vi "Hardware Out - NI 9758-1 (PFI-LS).vi"(8 "RT Data in":T1={"Refs"={"FPGA 1"=refnum, "FPGA 2"=refnum}, "EPT"={"MaxCAD"=0.0, "EPT Sim Enabled"=FALSE, "EPTxData"={"Sync"=FALSE, "CurrentCAD"=0.0, "Speed [RPM]"=0.0, "Config"=FALSE, "Rcvg Primary"=FALSE, "Stall"=FALSE, "Overflow"=FALSE, "Ratio Error"=FALSE, "Pattern Error"=FALSE, "Aux Warning"=FALSE, "Watchdog Error"=FALSE}}, "Raw Inputs"={"NI9752s"=[], "NI9757s"=[], "NI9411s"=[], "NI9220s"=[], "VRHalls"=[]}, "Control Inputs"={"Engine Speed [RPM]"=0.0, "Engine Status"=enum."STALLED", "Load Control \nMode"=enum."High-Idle Governor", "dt(s)"=0.0, "Number of Cylinders"=0, "Engine Displacement [cc]"=0.0, "StoichAFR"=0.0, "Q.LHV Fuel [kJ/kg]"=0.0, "BattV PSU [V]"=0.0, "12V PSU [V]"=0.0, "5V PSU [V]"=0.0, "Pedal Position [%]"=0.0, "Oil Pressure [kPa]"=0.0, "Oil Temp [C]"=0.0, "Oil Level [%]"=0.0, "Engine Coolant Temp (ECT) [C]"=0.0, "Engine Coolant Pressure [kPa]"=0.0, "Rail Pressure [bar]"=0.0, "Fuel Pressure [kPa]"=0.0, "Fuel Temp [C]"=0.0, "Vacuum Pressure [kPa]"=0.0, "Throttle Position [%]"=0.0, "Cam1 Advance [CAD]"=0.0, "Cam2 Advance [CAD]"=0.0, "Cam3 Advance [CAD]"=0.0, "Cam4 Advance [CAD]"=0.0, "CA50 Control Output [CAD]"=[], "CA50 Control Output Valid"=[], "Intake Air Temp (IAT) [C]"=0.0, "Barometric Air Pressure [kPa]"=0.0, "Intake Air Rel. Humidity [%]"=0.0, "Mass Air Flow (MAF) [kg/hr]"=0.0, "Turbo Inlet Air Pressure [kPa]"=0.0, "Turbo Inlet Air Temp [C]"=0.0, "Turbo Outlet Air Pressure [kPa]"=0.0, "Turbo Outlet Air Temp [C]"=0.0, "CAC Outlet Pressure [kPa]"=0.0, "CAC Outlet Temp [C]"=0.0, "Intake Manifold Pressure (MAP) [kPa]"=0.0, "Intake Manifold Temp (MAT) [C]"=0.0, "Exhaust Manifold Pressure [kPa]"=0.0, "Exhaust Manifold Temp [C]"=0.0, "HighP EGR Cooler Outlet Pressure [kPa]"=0.0, "HighP EGR Cooler Outlet Temp [C]"=0.0, "HighP EGR Differential Pressure [kPa]"=0.0, "HighP EGR Valve Position [%]"=0.0, "Turbo Outlet Exhaust Pressure [kPa]"=0.0, "Turbo Outlet Exhaust Temp [C]"=0.0, "VGT Position 1 [%]"=0.0, "VGT Position 2 [%]"=0.0, "Turbo Speed 1 [RPM]"=0.0, "Turbo Speed 2 [RPM]"=0.0, "LowP EGR Differential Pressure [kPa]"=0.0, "LowP EGR Valve Position [%]"=0.0, "UEGO1Lambda"=0.0, "UEGO1_Hot"=FALSE, "UEGO2Lambda"=0.0, "UEGO2_Hot"=FALSE, "Knock Intensity"=[], "Knock"=[]}, "Control Outputs"={"Pedal Desired [%]"=0.0, "MEP Desired [bar]"=0.0, "Fuel Desired [mg/cyc]"=0.0, "Intake MAP Desired [kPa]"=0.0, "Cam1 Advance Setpoint [CAD]"=0.0, "Cam2 Advance Setpoint [CAD]"=0.0, "HighP EGR Position Setpoint [%Open]"=0.0, "LowP EGR Position Setpoint [%Open]"=0.0, "Rail Pressure Setpoint [bar]"=0.0, "Wastegate1 Position Setpoint [%Open]"=0.0, "Wastegate2 Position Setpoint [%Open]"=0.0, "VGT1 Position Setpoint [%Open]"=0.0, "VGT2 Position Setpoint [%Open]"=0.0, "Throttle1 Position Setpoint [%Open]"=0.0, "Throttle2 Position Setpoint [%Open]"=0.0, "TurboBPV Position Setpoint [%Open]"=0.0, "Spark Dwells [msec]"=[], "Spark Timings [DBTDC]"=[], "PFI Quantities [mg/inj]"=[], "PFI Timings [DBTDC]"=[], "DI Quantities [mg/inj]"=[], "DI Timings [DBTDC]"=[]}, "Raw Outputs"={"9751-1"={"DI1"={"Window_Start (DBTDC)"=0.0, "Window_End (DBTDC)"=0.0, "Enable_Inj1"=FALSE, "Duration_Inj1 (msec)"=0.0, "Timing_Inj1 (DBTDC)"=0.0, "Enable_Inj2"=FALSE, "Duration_Inj2 (msec)"=0.0, "Timing_Inj2 (DBTDC)"=0.0, "Enable_Inj3"=FALSE, "Duration_Inj3 (msec)"=0.0, "Timing_Inj3 (DBTDC)"=0.0, "Enable_Inj4"=FALSE, "Duration_Inj4 (msec)"=0.0, "Timing_Inj4 (DBTDC)"=0.0, "Enable_Inj5"=FALSE, "Duration_Inj5 (msec)"=0.0, "Timing_Inj5 (DBTDC)"=0.0}, "DI2"={"Window_Start (DBTDC)"=0.0, "Window_End (DBTDC)"=0.0, "Enable_Inj1"=FALSE, "Duration_Inj1 (msec)"=0.0, "Timing_Inj1 (DBTDC)"=0.0, "Enable_Inj2"=FALSE, "Duration_Inj2 (msec)"=0.0, "Timing_Inj2 (DBTDC)"=0.0, "Enable_Inj3"=FALSE, "Duration_Inj3 (msec)"=0.0, "Timing_Inj3 (DBTDC)"=0.0, "Enable_Inj4"=FALSE, "Duration_Inj4 (msec)"=0.0, "Timing_Inj4 (DBTDC)"=0.0, "Enable_Inj5"=FALSE, "Duration_Inj5 (msec)"=0.0, "Timing_Inj5 (DBTDC)"=0.0}, "DI3"={"Window_Start (DBTDC)"=0.0, "Window_End (DBTDC)"=0.0, "Enable_Inj1"=FALSE, "Duration_Inj1 (msec)"=0.0, "Timing_Inj1 (DBTDC)"=0.0, "Enable_Inj2"=FALSE, "Duration_Inj2 (msec)"=0.0, "Timing_Inj2 (DBTDC)"=0.0, "Enable_Inj3"=FALSE, "Duration_Inj3 (msec)"=0.0, "Timing_Inj3 (DBTDC)"=0.0, "Enable_Inj4"=FALSE, "Duration_Inj4 (msec)"=0.0, "Timing_Inj4 (DBTDC)"=0.0, "Enable_Inj5"=FALSE, "Duration_Inj5 (msec)"=0.0, "Timing_Inj5 (DBTDC)"=0.0}}, "9751-2"={"DI1"={"Window_Start (DBTDC)"=0.0, "Window_End (DBTDC)"=0.0, "Enable_Inj1"=FALSE, "Duration_Inj1 (msec)"=0.0, "Timing_Inj1 (DBTDC)"=0.0, "Enable_Inj2"=FALSE, "Duration_Inj2 (msec)"=0.0, "Timing_Inj2 (DBTDC)"=0.0, "Enable_Inj3"=FALSE, "Duration_Inj3 (msec)"=0.0, "Timing_Inj3 (DBTDC)"=0.0, "Enable_Inj4"=FALSE, "Duration_Inj4 (msec)"=0.0, "Timing_Inj4 (DBTDC)"=0.0, "Enable_Inj5"=FALSE, "Duration_Inj5 (msec)"=0.0, "Timing_Inj5 (DBTDC)"=0.0}, "DI2"={"Window_Start (DBTDC)"=0.0, "Window_End (DBTDC)"=0.0, "Enable_Inj1"=FALSE, "Duration_Inj1 (msec)"=0.0, "Timing_Inj1 (DBTDC)"=0.0, "Enable_Inj2"=FALSE, "Duration_Inj2 (msec)"=0.0, "Timing_Inj2 (DBTDC)"=0.0, "Enable_Inj3"=FALSE, "Duration_Inj3 (msec)"=0.0, "Timing_Inj3 (DBTDC)"=0.0, "Enable_Inj4"=FALSE, "Duration_Inj4 (msec)"=0.0, "Timing_Inj4 (DBTDC)"=0.0, "Enable_Inj5"=FALSE, "Duration_Inj5 (msec)"=0.0, "Timing_Inj5 (DBTDC)"=0.0}, "DI3"={"Window_Start (DBTDC)"=0.0, "Window_End (DBTDC)"=0.0, "Enable_Inj1"=FALSE, "Duration_Inj1 (msec)"=0.0, "Timing_Inj1 (DBTDC)"=0.0, "Enable_Inj2"=FALSE, "Duration_Inj2 (msec)"=0.0, "Timing_Inj2 (DBTDC)"=0.0, "Enable_Inj3"=FALSE, "Duration_Inj3 (msec)"=0.0, "Timing_Inj3 (DBTDC)"=0.0, "Enable_Inj4"=FALSE, "Duration_Inj4 (msec)"=0.0, "Timing_Inj4 (DBTDC)"=0.0, "Enable_Inj5"=FALSE, "Duration_Inj5 (msec)"=0.0, "Timing_Inj5 (DBTDC)"=0.0}}, "9751-3"={"DI1"={"Window_Start (DBTDC)"=0.0, "Window_End (DBTDC)"=0.0, "Enable_Inj1"=FALSE, "Duration_Inj1 (msec)"=0.0, "Timing_Inj1 (DBTDC)"=0.0, "Enable_Inj2"=FALSE, "Duration_Inj2 (msec)"=0.0, "Timing_Inj2 (DBTDC)"=0.0, "Enable_Inj3"=FALSE, "Duration_Inj3 (msec)"=0.0, "Timing_Inj3 (DBTDC)"=0.0, "Enable_Inj4"=FALSE, "Duration_Inj4 (msec)"=0.0, "Timing_Inj4 (DBTDC)"=0.0, "Enable_Inj5"=FALSE, "Duration_Inj5 (msec)"=0.0, "Timing_Inj5 (DBTDC)"=0.0}, "DI2"={"Window_Start (DBTDC)"=0.0, "Window_End (DBTDC)"=0.0, "Enable_Inj1"=FALSE, "Duration_Inj1 (msec)"=0.0, "Timing_Inj1 (DBTDC)"=0.0, "Enable_Inj2"=FALSE, "Duration_Inj2 (msec)"=0.0, "Timing_Inj2 (DBTDC)"=0.0, "Enable_Inj3"=FALSE, "Duration_Inj3 (msec)"=0.0, "Timing_Inj3 (DBTDC)"=0.0, "Enable_Inj4"=FALSE, "Duration_Inj4 (msec)"=0.0, "Timing_Inj4 (DBTDC)"=0.0, "Enable_Inj5"=FALSE, "Duration_Inj5 (msec)"=0.0, "Timing_Inj5 (DBTDC)"=0.0}, "DI3"={"Window_Start (DBTDC)"=0.0, "Window_End (DBTDC)"=0.0, "Enable_Inj1"=FALSE, "Duration_Inj1 (msec)"=0.0, "Timing_Inj1 (DBTDC)"=0.0, "Enable_Inj2"=FALSE, "Duration_Inj2 (msec)"=0.0, "Timing_Inj2 (DBTDC)"=0.0, "Enable_Inj3"=FALSE, "Duration_Inj3 (msec)"=0.0, "Timing_Inj3 (DBTDC)"=0.0, "Enable_Inj4"=FALSE, "Duration_Inj4 (msec)"=0.0, "Timing_Inj4 (DBTDC)"=0.0, "Enable_Inj5"=FALSE, "Duration_Inj5 (msec)"=0.0, "Timing_Inj5 (DBTDC)"=0.0}}, "9751-4"={"DI1"={"Window_Start (DBTDC)"=0.0, "Window_End (DBTDC)"=0.0, "Enable_Inj1"=FALSE, "Duration_Inj1 (msec)"=0.0, "Timing_Inj1 (DBTDC)"=0.0, "Enable_Inj2"=FALSE, "Duration_Inj2 (msec)"=0.0, "Timing_Inj2 (DBTDC)"=0.0, "Enable_Inj3"=FALSE, "Duration_Inj3 (msec)"=0.0, "Timing_Inj3 (DBTDC)"=0.0, "Enable_Inj4"=FALSE, "Duration_Inj4 (msec)"=0.0, "Timing_Inj4 (DBTDC)"=0.0, "Enable_Inj5"=FALSE, "Duration_Inj5 (msec)"=0.0, "Timing_Inj5 (DBTDC)"=0.0}, "DI2"={"Window_Start (DBTDC)"=0.0, "Window_End (DBTDC)"=0.0, "Enable_Inj1"=FALSE, "Duration_Inj1 (msec)"=0.0, "Timing_Inj1 (DBTDC)"=0.0, "Enable_Inj2"=FALSE, "Duration_Inj2 (msec)"=0.0, "Timing_Inj2 (DBTDC)"=0.0, "Enable_Inj3"=FALSE, "Duration_Inj3 (msec)"=0.0, "Timing_Inj3 (DBTDC)"=0.0, "Enable_Inj4"=FALSE, "Duration_Inj4 (msec)"=0.0, "Timing_Inj4 (DBTDC)"=0.0, "Enable_Inj5"=FALSE, "Duration_Inj5 (msec)"=0.0, "Timing_Inj5 (DBTDC)"=0.0}, "DI3"={"Window_Start (DBTDC)"=0.0, "Window_End (DBTDC)"=0.0, "Enable_Inj1"=FALSE, "Duration_Inj1 (msec)"=0.0, "Timing_Inj1 (DBTDC)"=0.0, "Enable_Inj2"=FALSE, "Duration_Inj2 (msec)"=0.0, "Timing_Inj2 (DBTDC)"=0.0, "Enable_Inj3"=FALSE, "Duration_Inj3 (msec)"=0.0, "Timing_Inj3 (DBTDC)"=0.0, "Enable_Inj4"=FALSE, "Duration_Inj4 (msec)"=0.0, "Timing_Inj4 (DBTDC)"=0.0, "Enable_Inj5"=FALSE, "Duration_Inj5 (msec)"=0.0, "Timing_Inj5 (DBTDC)"=0.0}}, "9754-1"={"ESTTL 1"={"Timing (DBTDC)"=0.0, "Dwell (ms)"=0.0}, "ESTTL 2"={"Timing (DBTDC)"=0.0, "Dwell (ms)"=0.0}, "ESTTL 3"={"Timing (DBTDC)"=0.0, "Dwell (ms)"=0.0}, "ESTTL 4"={"Timing (DBTDC)"=0.0, "Dwell (ms)"=0.0}, "ESTTL 5"={"Timing (DBTDC)"=0.0, "Dwell (ms)"=0.0}, "ESTTL 6"={"Timing (DBTDC)"=0.0, "Dwell (ms)"=0.0}, "ESTTL 7"={"Timing (DBTDC)"=0.0, "Dwell (ms)"=0.0}, "ESTTL 8"={"Timing (DBTDC)"=0.0, "Dwell (ms)"=0.0}}, "9754-2"={"ESTTL 1"={"Timing (DBTDC)"=0.0, "Dwell (ms)"=0.0}, "ESTTL 2"={"Timing (DBTDC)"=0.0, "Dwell (ms)"=0.0}, "ESTTL 3"={"Timing (DBTDC)"=0.0, "Dwell (ms)"=0.0}, "ESTTL 4"={"Timing (DBTDC)"=0.0, "Dwell (ms)"=0.0}, "ESTTL 5"={"Timing (DBTDC)"=0.0, "Dwell (ms)"=0.0}, "ESTTL 6"={"Timing (DBTDC)"=0.0, "Dwell (ms)"=0.0}, "ESTTL 7"={"Timing (DBTDC)"=0.0, "Dwell (ms)"=0.0}, "ESTTL 8"={"Timing (DBTDC)"=0.0, "Dwell (ms)"=0.0}}, "9758-1"={"LS 1"={"Enable"=FALSE, "Freq [Hz]"=0.0, "DutyCyc [%]"=0.0}, "LS 2"={"Enable"=FALSE, "Freq [Hz]"=0.0, "DutyCyc [%]"=0.0}, "LS 3"={"Enable"=FALSE, "Freq [Hz]"=0.0, "DutyCyc [%]"=0.0}, "LS 4"={"Enable"=FALSE, "Freq [Hz]"=0.0, "DutyCyc [%]"=0.0}, "PFI 1"={"Position Mode"=FALSE, "Timing (DBTDC)"=0.0, "Pulse Width (ms)"=0.0}, "PFI 2"={"Position Mode"=FALSE, "Timing (DBTDC)"=0.0, "Pulse Width (ms)"=0.0}, "PFI 3"={"Position Mode"=FALSE, "Timing (DBTDC)"=0.0, "Pulse Width (ms)"=0.0}, "PFI 4"={"Position Mode"=FALSE, "Timing (DBTDC)"=0.0, "Pulse Width (ms)"=0.0}}, "9758-2"={"LS 1"={"Enable"=FALSE, "Freq [Hz]"=0.0, "DutyCyc [%]"=0.0}, "LS 2"={"Enable"=FALSE, "Freq [Hz]"=0.0, "DutyCyc [%]"=0.0}, "LS 3"={"Enable"=FALSE, "Freq [Hz]"=0.0, "DutyCyc [%]"=0.0}, "LS 4"={"Enable"=FALSE, "Freq [Hz]"=0.0, "DutyCyc [%]"=0.0}, "PFI 1"={"Position Mode"=FALSE, "Timing (DBTDC)"=0.0, "Pulse Width (ms)"=0.0}, "PFI 2"={"Position Mode"=FALSE, "Timing (DBTDC)"=0.0, "Pulse Width (ms)"=0.0}, "PFI 3"={"Position Mode"=FALSE, "Timing (DBTDC)"=0.0, "Pulse Width (ms)"=0.0}, "PFI 4"={"Position Mode"=FALSE, "Timing (DBTDC)"=0.0, "Pulse Width (ms)"=0.0}}, "9759-1"={"THR1-1 DC [%]"=0.0, "THR1-1 Setpoint [% Open]"=0.0, "THR1-2 DC [%]"=0.0, "THR1-2 Setpoint [% Open]"=0.0}}} {"Control Inputs"."Knock Intensity" format="%.2f"; "Control Inputs"."CA50 Control Output [CAD]" format="%.2f"; "Control Inputs"."Exhaust Manifold Temp [C]" format="%#_6f"; "Control Inputs"."UEGO2Lambda" format="%.2f"; "Control Inputs"."Intake Manifold Temp (MAT) [C]" format="%#_6f"; "Control Inputs"."UEGO1Lambda" format="%.2f"}, 11 "FPGA Ref":T3) -> ()   [LabVIEW 2015, in "ECS-RT.lvlib"]
uses:
  ECS-RT.lvlib
  Typedefs/FPGA Refs/Generic FPGA Ref.ctl
  Typedefs/RT Data.ctl
  Typedefs/FPGA Refs/FPGA Refs.ctl
  Typedefs/EPT/EPT Cluster.ctl
  <vilib>/Powertrain Controls/Device Drivers/Engine Position Tracking/EPTx/RevA/RT/Controls/EPTxData.ctl
  Typedefs/Raw Inputs/Raw Inputs.ctl
  Typedefs/Raw Inputs/NI9752.ctl
  Typedefs/Raw Inputs/PPWData.ctl
  Typedefs/Raw Inputs/NI9757.ctl
  Typedefs/Raw Inputs/NI9411.ctl
  Typedefs/Raw Inputs/NI9220.ctl
  Typedefs/Raw Inputs/VRHall.ctl
  Typedefs/Control Inputs/Control Inputs.ctl
  Typedefs/EPT/Engine Status.ctl
  Typedefs/MISC/Load Control Mode.ctl
  Typedefs/Control Outputs/Control Outputs.ctl
  Typedefs/Control Outputs/Injection Quantity.ctl
  Typedefs/Control Outputs/Injection Timing.ctl
  Typedefs/Raw Outputs/Raw Outputs.ctl
  Typedefs/Raw Outputs/NI9751.ctl
  Typedefs/Raw Outputs/DI.ctl
  Typedefs/Raw Outputs/NI9754.ctl
  Typedefs/Raw Outputs/ESTTL.ctl
  Typedefs/Raw Outputs/NI9758.ctl
  Typedefs/Raw Outputs/LS.ctl
  Typedefs/Raw Outputs/PFI.ctl
  Typedefs/Raw Outputs/NI9759.ctl
  <vilib>/Powertrain Controls/Device Drivers/Engine Position Tracking/EPTx/RevA/RT/Controls/EPTxFuelSparkControl.ctl
  <vilib>/Utility/error.llb/Error Cluster From Error Code.vi
  <vilib>/rvi/errors/niLvFpgaAdjustHostInterfaceError.vi
  Globals/TDC Globals.vi
  <vilib>/rvi/interface/nirviReadWriteControl/nirviReadWriteControl.xnode
  <vilib>/rvi/interface/Simulation/niFpgaSimulationCallBeginRW.vi
  <vilib>/Powertrain Controls/Device Drivers/Engine Position Tracking/EPTx/RevA/RT/EPTx - RevA - RT.lvlib
  NiFpgaLv.dll
  ECS-Shared.lvlib
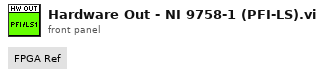
[diagram p1: front panel]
types:
  T1 = typedef "ECS-Shared.lvlib/RT Data.ctl" = cluster{"Refs":T2, "EPT":T4, "Raw Inputs":T6, "Control Inputs":T13, "Control Outputs":T16, "Raw Outputs":T19}
  T2 = typedef "ECS-Shared.lvlib/FPGA Refs.ctl" = cluster{"FPGA 1":T3, "FPGA 2":T3}
  T3 = typedef "ECS-Shared.lvlib/Generic FPGA Ref.ctl" = refnum<k20>
  T4 = typedef "ECS-Shared.lvlib/EPT Cluster.ctl" = cluster{"MaxCAD":sgl, "EPT Sim Enabled":bool, "EPTxData":T5}
  T5 = typedef "EPTx - RevA - RT.lvlib/EPTxData.ctl" = cluster{"Sync":bool, "CurrentCAD":sgl, "Speed [RPM]":sgl, "Config":bool, "Rcvg Primary":bool, "Stall":bool, "Overflow":bool, "Ratio Error":bool, "Pattern Error":bool, "Aux Warning":bool, "Watchdog Error":bool}
  T6 = typedef "ECS-Shared.lvlib/Raw Inputs.ctl" = cluster{"NI9752s":T7[], "NI9757s":T9[], "NI9411s":T10[], "NI9220s":T11[], "VRHalls":T12[]}
  T7 = typedef "ECS-Shared.lvlib/NI9752.ctl" = cluster{"Voltage [V]":sgl[], "Resistance [Ohm]":sgl[], "PPWData VR1":T8, "PPWData VR2":T8, "PPWData Hall1":T8, "PPWData Hall2":T8}
  T8 = typedef "ECS-Shared.lvlib/PPWData.ctl" = cluster{"Period":u32, "PulseWidth":u32, "Stopped":bool}
  T9 = typedef "ECS-Shared.lvlib/NI9757.ctl" = cluster{"UEGO1":cluster{"Lambda":sgl, "Phi":sgl, "AF_Ratio":sgl, "Ip":sgl, "Temp":sgl, "Hot":bool}, "UEGO2":cluster{"Lambda":sgl, "Phi":sgl, "AF_Ratio":sgl, "Ip":sgl, "Temp":sgl, "Hot":bool}, "EGO1":cluster{"Status":enum16{"COLD SENSOR", "FOULED SENSOR", "RICH", "LEAN"}, "SensorV":sgl}, "EGO2":cluster{"Status":enum16{"COLD SENSOR", "FOULED SENSOR", "RICH", "LEAN"}, "SensorV":sgl}, "EGO3":cluster{"Status":enum16{"COLD SENSOR", "FOULED SENSOR", "RICH", "LEAN"}, "SensorV":sgl}, "EGO4":cluster{"Status":enum16{"COLD SENSOR", "FOULED SENSOR", "RICH", "LEAN"}, "SensorV":sgl}}
  T10 = typedef "ECS-Shared.lvlib/NI9411.ctl" = cluster{"PPWData 0":T8, "PPWData 1":T8, "PPWData 2":T8, "PPWData 3":T8, "PPWData 4":T8, "PPWData 5":T8}
  T11 = typedef "ECS-Shared.lvlib/NI9220.ctl" = cluster{"AI 0":sgl, "AI 1":sgl, "AI 2":sgl, "AI 3":sgl, "AI 4":sgl, "AI 5":sgl, "AI 6":sgl, "AI 7":sgl, "AI 8":sgl, "AI 9":sgl, "AI 10":sgl, "AI 11":sgl, "AI 12":sgl, "AI 13":sgl, "AI 14":sgl, "AI 15":sgl}
  T12 = typedef "ECS-Shared.lvlib/VRHall.ctl" = cluster{"PPWData 0":T8, "PPWData 1":T8, "PPWData 2":T8, "PPWData 3":T8, "PPWData 4":T8, "PPWData 5":T8}
  T13 = typedef "ECS-Shared.lvlib/Control Inputs.ctl" = cluster{"Engine Speed [RPM]":sgl, "Engine Status":T14, "Load Control \nMode":T15, "dt(s)":sgl, "Number of Cylinders":u8, "Engine Displacement [cc]":sgl, "StoichAFR":sgl, "Q.LHV Fuel [kJ/kg]":sgl, "BattV PSU [V]":sgl, "12V PSU [V]":sgl, "5V PSU [V]":sgl, "Pedal Position [%]":sgl, "Oil Pressure [kPa]":sgl, "Oil Temp [C]":sgl, "Oil Level [%]":sgl, "Engine Coolant Temp (ECT) [C]":sgl, "Engine Coolant Pressure [kPa]":sgl, "Rail Pressure [bar]":sgl, "Fuel Pressure [kPa]":sgl, "Fuel Temp [C]":sgl, "Vacuum Pressure [kPa]":sgl, "Throttle Position [%]":sgl, "Cam1 Advance [CAD]":sgl, "Cam2 Advance [CAD]":sgl, "Cam3 Advance [CAD]":sgl, "Cam4 Advance [CAD]":sgl, "CA50 Control Output [CAD]":sgl[], "CA50 Control Output Valid":bool[], "Intake Air Temp (IAT) [C]":sgl, "Barometric Air Pressure [kPa]":sgl, "Intake Air Rel. Humidity [%]":sgl, "Mass Air Flow (MAF) [kg/hr]":sgl, "Turbo Inlet Air Pressure [kPa]":sgl, "Turbo Inlet Air Temp [C]":sgl, "Turbo Outlet Air Pressure [kPa]":sgl, "Turbo Outlet Air Temp [C]":sgl, "CAC Outlet Pressure [kPa]":sgl, "CAC Outlet Temp [C]":sgl, "Intake Manifold Pressure (MAP) [kPa]":sgl, "Intake Manifold Temp (MAT) [C]":sgl, "Exhaust Manifold Pressure [kPa]":sgl, "Exhaust Manifold Temp [C]":sgl, "HighP EGR Cooler Outlet Pressure [kPa]":sgl, "HighP EGR Cooler Outlet Temp [C]":sgl, "HighP EGR Differential Pressure [kPa]":sgl, "HighP EGR Valve Position [%]":sgl, "Turbo Outlet Exhaust Pressure [kPa]":sgl, "Turbo Outlet Exhaust Temp [C]":sgl, "VGT Position 1 [%]":sgl, "VGT Position 2 [%]":sgl, "Turbo Speed 1 [RPM]":sgl, "Turbo Speed 2 [RPM]":sgl, "LowP EGR Differential Pressure [kPa]":sgl, "LowP EGR Valve Position [%]":sgl, "UEGO1Lambda":sgl, "UEGO1_Hot":bool, "UEGO2Lambda":sgl, "UEGO2_Hot":bool, "Knock Intensity":sgl[], "Knock":bool[]}
  T14 = typedef "ECS-Shared.lvlib/Engine Status.ctl" = enum16{"OFF", "STALLED", "CRANKING", "RUNNING", "ACCEL", "DECEL", "SAFE"}
  T15 = typedef "ECS-Shared.lvlib/Load Control Mode.ctl" = enum16{"No Governor", "Low-Idle Governor", "High-Idle Governor"}
  T16 = typedef "ECS-Shared.lvlib/Control Outputs.ctl" = cluster{"Pedal Desired [%]":sgl, "MEP Desired [bar]":sgl, "Fuel Desired [mg/cyc]":sgl, "Intake MAP Desired [kPa]":sgl, "Cam1 Advance Setpoint [CAD]":sgl, "Cam2 Advance Setpoint [CAD]":sgl, "HighP EGR Position Setpoint [%Open]":sgl, "LowP EGR Position Setpoint [%Open]":sgl, "Rail Pressure Setpoint [bar]":sgl, "Wastegate1 Position Setpoint [%Open]":sgl, "Wastegate2 Position Setpoint [%Open]":sgl, "VGT1 Position Setpoint [%Open]":sgl, "VGT2 Position Setpoint [%Open]":sgl, "Throttle1 Position Setpoint [%Open]":sgl, "Throttle2 Position Setpoint [%Open]":sgl, "TurboBPV Position Setpoint [%Open]":sgl, "Spark Dwells [msec]":sgl[], "Spark Timings [DBTDC]":sgl[], "PFI Quantities [mg/inj]":sgl[], "PFI Timings [DBTDC]":sgl[], "DI Quantities [mg/inj]":T17[], "DI Timings [DBTDC]":T18[]}
  T17 = typedef "ECS-Shared.lvlib/Injection Quantity.ctl" = cluster{"Pilot1Quantity [mg/inj]":sgl, "Pilot2Quantity [mg/inj]":sgl, "MainQuantity [mg/inj]":sgl, "Post1Quantity [mg/inj]":sgl, "Post2Quantity [mg/inj]":sgl}
  T18 = typedef "ECS-Shared.lvlib/Injection Timing.ctl" = cluster{"Pilot1SOI [DBTDC]":sgl, "Pilot2SOI [DBTDC]":sgl, "MainSOI [DBTDC]":sgl, "Post1SOI [DBTDC]":sgl, "Post2SOI [DBTDC]":sgl}
  T19 = typedef "ECS-Shared.lvlib/Raw Outputs.ctl" = cluster{"9751-1":T20, "9751-2":T20, "9751-3":T20, "9751-4":T20, "9754-1":T22, "9754-2":T22, "9758-1":T24, "9758-2":T24, "9759-1":T27}
  T20 = typedef "ECS-Shared.lvlib/NI9751.ctl" = cluster{"DI1":T21, "DI2":T21, "DI3":T21}
  T21 = typedef "ECS-Shared.lvlib/DI.ctl" = cluster{"Window_Start (DBTDC)":sgl, "Window_End (DBTDC)":sgl, "Enable_Inj1":bool, "Duration_Inj1 (msec)":sgl, "Timing_Inj1 (DBTDC)":sgl, "Enable_Inj2":bool, "Duration_Inj2 (msec)":sgl, "Timing_Inj2 (DBTDC)":sgl, "Enable_Inj3":bool, "Duration_Inj3 (msec)":sgl, "Timing_Inj3 (DBTDC)":sgl, "Enable_Inj4":bool, "Duration_Inj4 (msec)":sgl, "Timing_Inj4 (DBTDC)":sgl, "Enable_Inj5":bool, "Duration_Inj5 (msec)":sgl, "Timing_Inj5 (DBTDC)":sgl}
  T22 = typedef "ECS-Shared.lvlib/NI9754.ctl" = cluster{"ESTTL 1":T23, "ESTTL 2":T23, "ESTTL 3":T23, "ESTTL 4":T23, "ESTTL 5":T23, "ESTTL 6":T23, "ESTTL 7":T23, "ESTTL 8":T23}
  T23 = typedef "ECS-Shared.lvlib/ESTTL.ctl" = cluster{"Timing (DBTDC)":sgl, "Dwell (ms)":sgl}
  T24 = typedef "ECS-Shared.lvlib/NI9758.ctl" = cluster{"LS 1":T25, "LS 2":T25, "LS 3":T25, "LS 4":T25, "PFI 1":T26, "PFI 2":T26, "PFI 3":T26, "PFI 4":T26}
  T25 = typedef "ECS-Shared.lvlib/LS.ctl" = cluster{"Enable":bool, "Freq [Hz]":sgl, "DutyCyc [%]":sgl}
  T26 = typedef "ECS-Shared.lvlib/PFI.ctl" = cluster{"Position Mode":bool, "Timing (DBTDC)":sgl, "Pulse Width (ms)":sgl}
  T27 = typedef "ECS-Shared.lvlib/NI9759.ctl" = cluster{"THR1-1 DC [%]":sgl, "THR1-1 Setpoint [% Open]":sgl, "THR1-2 DC [%]":sgl, "THR1-2 Setpoint [% Open]":sgl}
  T28 = typedef "EPTx - RevA - RT.lvlib/EPTxFuelSparkControl.ctl" = cluster{"Enable":bool, "Window Start [DBTDC]":sgl, "Window End [DBTDC]":sgl, "Timing [DBTDC]":sgl, "Duration [ms]":sgl, "Timing Mode (SA=F, EA=T)":bool, "Min Duration [ms]":sgl, "Max Duration [ms]":sgl}
  T29 = cluster{"LS1Period":u32, "LS1PulseWidth":u32, "LS2Period":u32, "LS2PulseWidth":u32, "LS3Period":u32, "LS3PulseWidth":u32, "LS4Period":u32, "LS4PulseWidth":u32}
  T30 = cluster{"ModuleEnable":bool, "LS1Enable":bool, "LS2Enable":bool, "LS3Enable":bool, "LS4Enable":bool, "PFI1Enable":bool, "PFI2Enable":bool, "PFI3Enable":bool, "PFI4Enable":bool, "RecircAlways1":bool, "RecircAlways2":bool, "RecircAlways3":bool, "RecircAlways4":bool, "Phase1FirstPeak1":bool, "Phase1FirstPeak2":bool, "Phase1FirstPeak3":bool, "Phase1FirstPeak4":bool, "OneShotSelect":enum8{"DISABLED", "PFI 1", "PFI 2", "PFI 3", "PFI 4"}, "One Shot Time (msec)":sgl, "OneShot":bool, "Fault_ClrSig":bool}
  T31 = cluster{"IPhaseCurrent":u16, "IPhaseDuration":u16}[]
  T32 = typedef "EPTx - RevA - FPGA.lvlib/EPTxFuelSparkControl.ctl" = cluster{"Enable":bool, "Window Start [CAD]":fxp<+,18,11>, "Window End [CAD]":fxp<+,18,11>, "Timing [CAD]":fxp<+,18,11>, "Duration [ms]":fxp<+/-,22,9>}
  T33 = cluster{"ModuleEnable":bool, "WatchdogIn":bool, "OneShotSelect":enum8{"DISABLED", "PFI 1", "PFI 2", "PFI 3", "PFI 4"}, "OneShotTime":u32, "OneShot":bool, "Control":u16, "HostMode":u8, "HostCommand":u32, "Fault_ClrSig":bool}
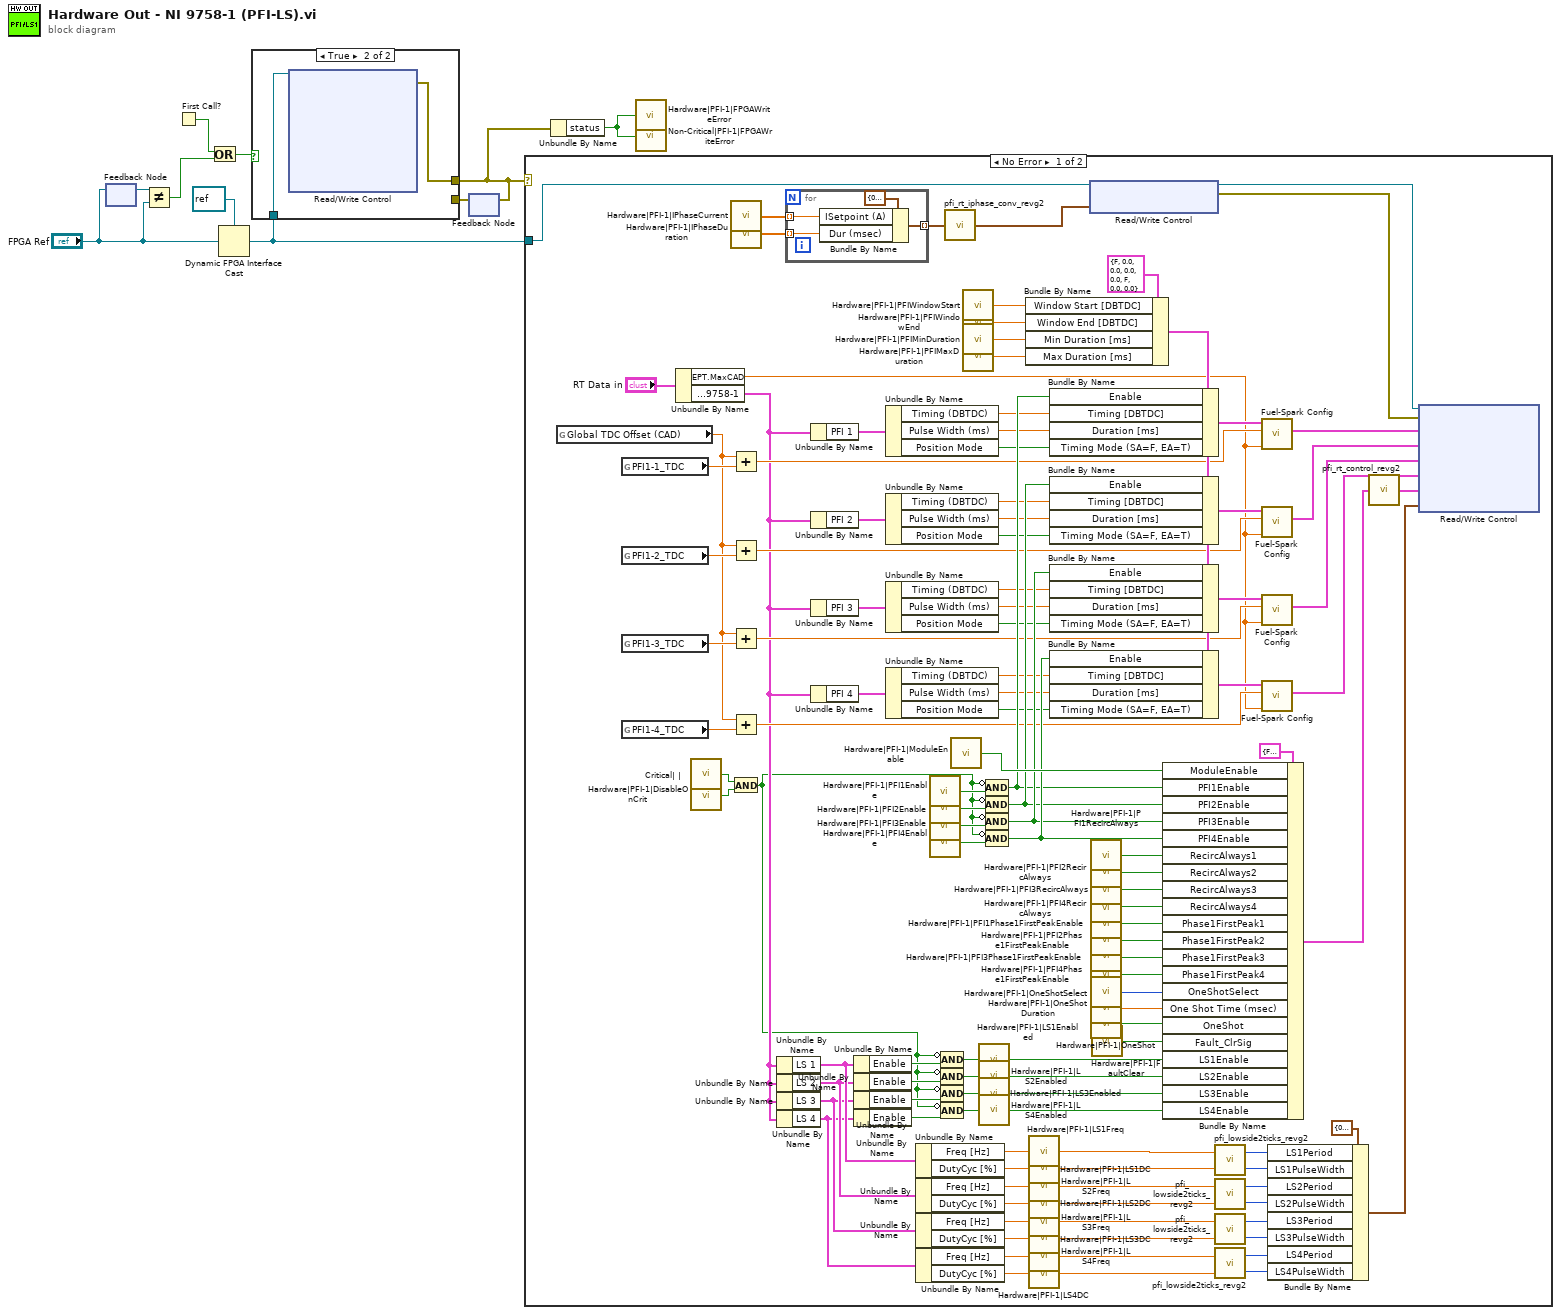
[diagram p0: block diagram]
diagram:
  n1 = feedback #1() -> (w7:T3)  [unwired: 1 in]
  n2 = feedback-in #1("FPGA Ref") -> ()
  n3 = Not Equal?(x=w7, y="FPGA Ref") -> (x != y?=w6:bool)
  n4 = First Call?() -> (First Call?: T/F=w8:bool)
  n5 = Or(x=w8, y=w6) -> (x .or. y?=w9:bool)
  n6 = Dynamic FPGA Interface Cast(Session In=refnum<k20> refnum ("NI 9758-1 (PFI-LS)"), Type="FPGA Ref") -> (Session Out=w3:refnum<k20>)
  n7 = feedback #2() -> (w10:errorcluster)  [unwired: 1 in]
  n8 = case shown="True" w9 {
    tunnel: [w11 w13] -> w2
    tunnel: w10 -> [w11 _]
    tunnel: w3 -> [_ w12]
    frame False {
    }
    frame True {
      n9 = xnode "Read/Write Control"("FPGA VI Reference In"=w12) -> ("error out"=w13:errorcluster)  [unwired: 8 in, 1 out]
    }
  }
  n10 = feedback-in #2(w2) -> ()
  n11 = case shown="No Error" w2 {
    tunnel: w3 -> [w63 _]
    frame No Error {
      n12 = global read "TDC Globals.vi" "Global TDC Offset (CAD)"() -> (w62:sgl)
      n13 = global read "TDC Globals.vi" "PFI1-1_TDC"() -> (w66:sgl)
      n14 = global read "TDC Globals.vi" "PFI1-2_TDC"() -> (w67:sgl)
      n15 = global read "TDC Globals.vi" "PFI1-3_TDC"() -> (w68:sgl)
      n16 = global read "TDC Globals.vi" "PFI1-4_TDC"() -> (w69:sgl)
      n17 = Unbundle By Name("RT Data in") -> ("EPT.MaxCAD"=w22:sgl, "Raw Outputs.9758-1"=w21:T24)
      n18 = call "Critical| |"() -> ("Fault"=w16:bool)  [unwired: 2 in]
      n19 = call "Hardware|PFI-1|DisableOnCrit"() -> ("Value"=w15:bool)
      n20 = call "Hardware|PFI-1|IPhaseCurrent"() -> ("Value"=w77:sgl[])
      n21 = call "Hardware|PFI-1|IPhaseDuration"() -> ("Value"=w78:sgl[])
      n22 = Add(x=w62, y=w66) -> (x+y=w31:sgl)
      n23 = Add(x=w62, y=w67) -> (x+y=w30:sgl)
      n24 = Add(x=w62, y=w68) -> (x+y=w29:sgl)
      n25 = Add(x=w62, y=w69) -> (x+y=w28:sgl)
      n26 = And(x=w16, y=w15) -> (x .and. y?=w14:bool)
      n27 = Unbundle By Name(w21) -> ("LS 1"=w20:T25)
      n28 = Unbundle By Name(w21) -> ("LS 2"=w19:T25)
      n29 = Unbundle By Name(w21) -> ("LS 3"=w18:T25)
      n30 = Unbundle By Name(w21) -> ("LS 4"=w17:T25)
      n31 = for {
        tunnel: w77 -> [w123] mode=indexing
        tunnel: w78 -> [w122] mode=indexing
        tunnel: [w121] -> w79 mode=indexing
        n32 = Bundle By Name(cluster=cluster{"ISetpoint (A)":sgl, "Dur (msec)":sgl} {"ISetpoint (A)"=0.0, "Dur (msec)"=0.0} ("IPhaseInterface"), "ISetpoint (A)"=w123, "Dur (msec)"=w122) -> (w121:cluster{"ISetpoint (A)":sgl, "Dur (msec)":sgl})
      }
      n33 = Unbundle By Name(w21) -> ("PFI 1"=w27:T26)
      n34 = Unbundle By Name(w21) -> ("PFI 2"=w25:T26)
      n35 = Unbundle By Name(w21) -> ("PFI 3"=w24:T26)
      n36 = Unbundle By Name(w21) -> ("PFI 4"=w23:T26)
      n37 = Unbundle By Name(w20) -> ("Enable"=w118:bool)
      n38 = Unbundle By Name(w19) -> ("Enable"=w119:bool)
      n39 = Unbundle By Name(w18) -> ("Enable"=w95:bool)
      n40 = Unbundle By Name(w17) -> ("Enable"=w94:bool)
      n41 = Unbundle By Name(w27) -> ("Timing (DBTDC)"=w43:sgl, "Pulse Width (ms)"=w42:sgl, "Position Mode"=w41:bool)
      n42 = Unbundle By Name(w25) -> ("Timing (DBTDC)"=w40:sgl, "Pulse Width (ms)"=w39:sgl, "Position Mode"=w38:bool)
      n43 = Unbundle By Name(w24) -> ("Timing (DBTDC)"=w37:sgl, "Pulse Width (ms)"=w36:sgl, "Position Mode"=w35:bool)
      n44 = Unbundle By Name(w23) -> ("Timing (DBTDC)"=w34:sgl, "Pulse Width (ms)"=w33:sgl, "Position Mode"=w32:bool)
      n45 = Unbundle By Name(w20) -> ("Freq [Hz]"=w87:sgl, "DutyCyc [%]"=w86:sgl)
      n46 = Unbundle By Name(w19) -> ("Freq [Hz]"=w85:sgl, "DutyCyc [%]"=w84:sgl)
      n47 = Unbundle By Name(w18) -> ("Freq [Hz]"=w83:sgl, "DutyCyc [%]"=w82:sgl)
      n48 = Unbundle By Name(w17) -> ("Freq [Hz]"=w81:sgl, "DutyCyc [%]"=w80:sgl)
      n49 = call "Hardware|PFI-1|PFI1Enable"() -> ("Value"=w113:bool)
      n50 = call "Hardware|PFI-1|PFI2Enable"() -> ("Value"=w114:bool)
      n51 = call "Hardware|PFI-1|PFI3Enable"() -> ("Value"=w115:bool)
      n52 = call "Hardware|PFI-1|PFI4Enable"() -> ("Value"=w116:bool)
      n53 = Compound Arithmetic op=AND(invert w14, w118) -> (w75:bool)
      n54 = Compound Arithmetic op=AND(invert w14, w119) -> (w74:bool)
      n55 = Compound Arithmetic op=AND(invert w14, w95) -> (w73:bool)
      n56 = Compound Arithmetic op=AND(invert w14, w94) -> (w72:bool)
      n57 = call <vilib>:"pfi_rt_iphase_conv_revg2.vi"("IPhaseArrayIn"=w79) -> ("IPhaseArrayOut"=w76:T31)
      n58 = call "Hardware|PFI-1|ModuleEnable"() -> ("Value"=w117:bool)
      n59 = call "Hardware|PFI-1|PFIWindowStart"() -> ("Value"=w48:sgl)
      n60 = call "Hardware|PFI-1|PFIWindowEnd"() -> ("Value"=w47:sgl)
      n61 = call "Hardware|PFI-1|PFIMinDuration"() -> ("Value"=w45:sgl)
      n62 = call "Hardware|PFI-1|PFIMaxDuration"() -> ("Value"=w44:sgl)
      n63 = call "Hardware|PFI-1|LS1Enabled"("Value"=w75) -> ()
      n64 = call "Hardware|PFI-1|LS2Enabled"("Value"=w74) -> ()
      n65 = call "Hardware|PFI-1|LS3Enabled"("Value"=w73) -> ()
      n66 = call "Hardware|PFI-1|LS4Enabled"("Value"=w72) -> ()
      n67 = Compound Arithmetic op=AND(invert w14, w113) -> (w50:bool)
      n68 = Compound Arithmetic op=AND(invert w14, w114) -> (w51:bool)
      n69 = Compound Arithmetic op=AND(invert w14, w115) -> (w52:bool)
      n70 = Compound Arithmetic op=AND(invert w14, w116) -> (w53:bool)
      n71 = Bundle By Name(cluster=T28 {"Enable"=FALSE, "Window Start [DBTDC]"=0.0, "Window End [DBTDC]"=0.0, "Timing [DBTDC]"=0.0, "Duration [ms]"=0.0, "Timing Mode (SA=F, EA=T)"=FALSE, "Min Duration [ms]"=0.0, "Max Duration [ms]"=0.0} ("Fuel-Spark Control"), "Window Start [DBTDC]"=w48, "Window End [DBTDC]"=w47, "Min Duration [ms]"=w45, "Max Duration [ms]"=w44) -> (w46:T28)
      n72 = call "Hardware|PFI-1|LS1Freq"("Value"=w87) -> ()
      n73 = call "Hardware|PFI-1|LS1DC"("Value"=w86) -> ()
      n74 = call "Hardware|PFI-1|LS2Freq"("Value"=w85) -> ()
      n75 = call "Hardware|PFI-1|LS2DC"("Value"=w84) -> ()
      n76 = call "Hardware|PFI-1|LS3Freq"("Value"=w83) -> ()
      n77 = call "Hardware|PFI-1|LS3DC"("Value"=w82) -> ()
      n78 = call "Hardware|PFI-1|LS4Freq"("Value"=w81) -> ()
      n79 = call "Hardware|PFI-1|LS4DC"("Value"=w80) -> ()
      n80 = Bundle By Name(cluster=w46, "Enable"=w50, "Timing [DBTDC]"=w43, "Duration [ms]"=w42, "Timing Mode (SA=F, EA=T)"=w41) -> (w57:T28)
      n81 = Bundle By Name(cluster=w46, "Enable"=w51, "Timing [DBTDC]"=w40, "Duration [ms]"=w39, "Timing Mode (SA=F, EA=T)"=w38) -> (w56:T28)
      n82 = Bundle By Name(cluster=w46, "Enable"=w52, "Timing [DBTDC]"=w37, "Duration [ms]"=w36, "Timing Mode (SA=F, EA=T)"=w35) -> (w55:T28)
      n83 = Bundle By Name(cluster=w46, "Enable"=w53, "Timing [DBTDC]"=w34, "Duration [ms]"=w33, "Timing Mode (SA=F, EA=T)"=w32) -> (w54:T28)
      n84 = xnode "Read/Write Control"("FPGA VI Reference In"=w63, "PFI-1.IPhaseInterface"=w76) -> ("FPGA VI Reference Out"=w65:refnum<k20>, "error out"=w64:errorcluster)  [unwired: 1 in]
      n85 = call "Hardware|PFI-1|PFI1RecircAlways"() -> ("Value"=w111:bool)
      n86 = call "Hardware|PFI-1|PFI2RecircAlways"() -> ("Value"=w110:bool)
      n87 = call "Hardware|PFI-1|PFI3RecircAlways"() -> ("Value"=w109:bool)
      n88 = call "Hardware|PFI-1|PFI4RecircAlways"() -> ("Value"=w108:bool)
      n89 = call "Hardware|PFI-1|PFI1Phase1FirstPeakEnable"() -> ("Value"=w107:bool)
      n90 = call "Hardware|PFI-1|PFI2Phase1FirstPeakEnable"() -> ("Value"=w106:bool)
      n91 = call "Hardware|PFI-1|PFI3Phase1FirstPeakEnable"() -> ("Value"=w105:bool)
      n92 = call "Hardware|PFI-1|PFI4Phase1FirstPeakEnable"() -> ("Value"=w104:bool)
      n93 = call "Hardware|PFI-1|OneShotSelect"() -> ("Value"=w101:u32)
      n94 = call "Hardware|PFI-1|OneShotDuration"() -> ("Value"=w100:sgl)
      n95 = call "Hardware|PFI-1|OneShot"() -> ("Value"=w103:bool)
      n96 = call "Hardware|PFI-1|FaultClear"() -> ("Value"=w102:bool)
      n97 = Bundle By Name(cluster=T30 {"ModuleEnable"=FALSE, "LS1Enable"=FALSE, "LS2Enable"=FALSE, "LS3Enable"=FALSE, "LS4Enable"=FALSE, "PFI1Enable"=FALSE, "PFI2Enable"=FALSE, "PFI3Enable"=FALSE, "PFI4Enable"=FALSE, "RecircAlways1"=FALSE, "RecircAlways2"=FALSE, "RecircAlways3"=FALSE, "RecircAlways4"=FALSE, "Phase1FirstPeak1"=FALSE, "Phase1FirstPeak2"=FALSE, "Phase1FirstPeak3"=FALSE, "Phase1FirstPeak4"=FALSE, "OneShotSelect"=enum."DISABLED", "One Shot Time (msec)"=5.0, "OneShot"=FALSE, "Fault_ClrSig"=FALSE} ("PFIControl"), "ModuleEnable"=w117, "PFI1Enable"=w50, "PFI2Enable"=w51, "PFI3Enable"=w52, "PFI4Enable"=w53, "RecircAlways1"=w111, "RecircAlways2"=w110, "RecircAlways3"=w109, "RecircAlways4"=w108, "Phase1FirstPeak1"=w107, "Phase1FirstPeak2"=w106, "Phase1FirstPeak3"=w105, "Phase1FirstPeak4"=w104, "OneShotSelect"=w101, "One Shot Time (msec)"=w100, "OneShot"=w103, "Fault_ClrSig"=w102, "LS1Enable"=w75, "LS2Enable"=w74, "LS3Enable"=w73, "LS4Enable"=w72) -> (w70:T30)
      n98 = call <vilib>:"pfi_lowside2ticks_revg2.vi"("DutyCycle (%)"=w86, "Frequency (Hz)"=w87) -> ("LSPulseWidthTicks"=w97:u32, "LSPeriodTicks"=w98:u32)
      n99 = call <vilib>:"pfi_lowside2ticks_revg2.vi"("DutyCycle (%)"=w84, "Frequency (Hz)"=w85) -> ("LSPulseWidthTicks"=w92:u32, "LSPeriodTicks"=w93:u32)
      n100 = call <vilib>:"pfi_lowside2ticks_revg2.vi"("DutyCycle (%)"=w82, "Frequency (Hz)"=w83) -> ("LSPulseWidthTicks"=w90:u32, "LSPeriodTicks"=w91:u32)
      n101 = call <vilib>:"pfi_lowside2ticks_revg2.vi"("DutyCycle (%)"=w80, "Frequency (Hz)"=w81) -> ("LSPulseWidthTicks"=w88:u32, "LSPeriodTicks"=w89:u32)
      n102 = call <vilib>:"Fuel-Spark Config.vi"("Max CAD"=w22, "Cylinder TDC [Absolute CAD]"=w31, "Fuel-Spark Control"=w57) -> ("Fuel-Spark Control"=w61:T32)  [unwired: 8 in]
      n103 = call <vilib>:"Fuel-Spark Config.vi"("Max CAD"=w22, "Cylinder TDC [Absolute CAD]"=w30, "Fuel-Spark Control"=w56) -> ("Fuel-Spark Control"=w60:T32)  [unwired: 8 in]
      n104 = call <vilib>:"Fuel-Spark Config.vi"("Max CAD"=w22, "Cylinder TDC [Absolute CAD]"=w29, "Fuel-Spark Control"=w55) -> ("Fuel-Spark Control"=w59:T32)  [unwired: 8 in]
      n105 = call <vilib>:"Fuel-Spark Config.vi"("Max CAD"=w22, "Cylinder TDC [Absolute CAD]"=w28, "Fuel-Spark Control"=w54) -> ("Fuel-Spark Control"=w58:T32)  [unwired: 8 in]
      n106 = Bundle By Name(cluster=T29 {"LS1Period"=0, "LS1PulseWidth"=0, "LS2Period"=0, "LS2PulseWidth"=0, "LS3Period"=0, "LS3PulseWidth"=0, "LS4Period"=0, "LS4PulseWidth"=0} ("PFI1.LowsidePWM"), "LS1Period"=w98, "LS1PulseWidth"=w97, "LS2Period"=w93, "LS2PulseWidth"=w92, "LS3Period"=w91, "LS3PulseWidth"=w90, "LS4Period"=w89, "LS4PulseWidth"=w88) -> (w96:T29)
      n107 = call <vilib>:"pfi_rt_control_revg2.vi"("PFIControl"=w70) -> ("PFIControlToFPGA"=w71:T33)  [unwired: 4 in]
      n108 = xnode "Read/Write Control"("FPGA VI Reference In"=w65, "error in"=w64, "PFI-1.FuelControl 1"=w61, "PFI-1.FuelControl 2"=w60, "PFI-1.FuelControl 3"=w59, "PFI-1.FuelControl 4"=w58, "PFI-1.Control"=w71, "PFI-1.LowsidePWM"=w96) -> ()  [unwired: 2 out]
    }
    frame Error {
    }
  }
  n109 = Unbundle By Name(w2) -> ("status"=w1:bool)
  n110 = call "Hardware|PFI-1|FPGAWriteError"("Value"=w1) -> ()
  n111 = call "Non-Critical|PFI-1|FPGAWriteError"("Fault"=w1) -> ()  [unwired: 2 in]
